vi "Submit Goal.vi"(8 "error in (no error)":errorcluster, 10 "Objective(s)":dbl[](array[numeric]) format="%#_13g", 11 "Generic Optimizer in":refnum<class "Generic Optimizer.lvclass">) -> (0 "error out":errorcluster, 3 "Generic Optimizer out":refnum<class "Generic Optimizer.lvclass">)   [LabVIEW 2020, in "RxnRover.lvlib" / "Generic Optimizer.lvclass"]
uses:
  Generic Optimizer.lvclass
  Generic Optimizer.lvclass/Generic Optimizer.ctl
  <userlib>/RxnRover/DynamicReentrant/Dynamic Reentrant.lvlib
  <vilib>/ErrorRing/Error Ring.xnode
  <vilib>/Utility/error.llb/Error Cluster From Error Code.vi
  Controller/Generic Plugin.lvclass
  C:/Users/zachc/programs/rxnrover_workspace/projects/rxnrover_exe/rxnrover/src/RxnRover/Plugin Servers/Controller/Generic Plugin.lvclass
  C:/Users/zachc/programs/rxnrover_workspace/projects/rxnrover_exe/rxnrover/src/RxnRover/Plugin Servers/Generic Optimizer/Generic Optimizer.lvclass
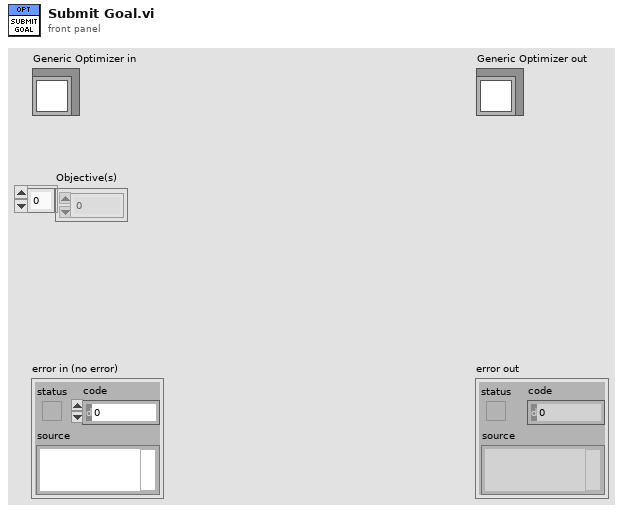
[diagram p1: front panel]
types:
  T1 = typedef "Dynamic Reentrant.lvlib/Message.ctl" = cluster{"Source":string, "Destination":string, "Time Stamp":timestamp, "Command":string, "Data":variant}
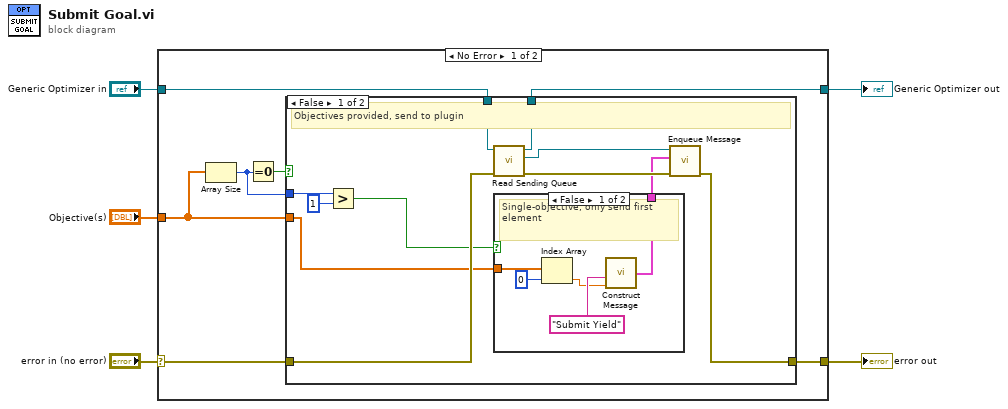
[diagram p0: block diagram]
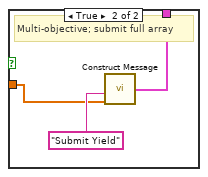
[diagram p2: hidden frame]
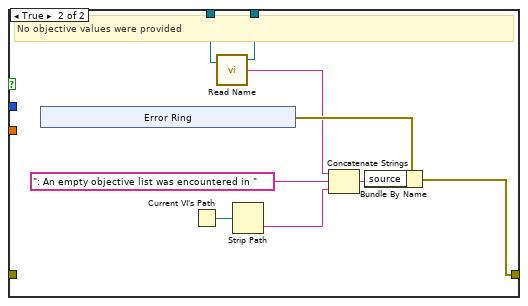
[diagram p3: hidden frame]
diagram:
  n1 = case shown="No Error" "error in (no error)" {
    selector: "error in (no error)" -> [w12 w46]
    tunnel: [w9 w46] -> w4
    tunnel: [w10 w45] -> w2
    tunnel: "Generic Optimizer in" -> [w11 w45]
    tunnel: "Objective(s)" -> [w7 _]
    frame No Error {
      n2 = Array Size(array=w7) -> (size(s)=w6:i32)
      n3 = Equal To 0?(x=w6) -> (x = 0?=w8:bool)
      n4 = case shown="False" w8 {
        tunnel: w12 -> [w23 _]
        tunnel: w11 -> [w22 w40]
        tunnel: [w21 w38] -> w10
        tunnel: [w17 w32] -> w9
        tunnel: w7 -> [w13 _]
        tunnel: w6 -> [w16 _]
        frame False {
          # "Objectives provided, send to plugin"
          n5 = Greater?(x=w16, y=1) -> (0:w14:bool)
          n6 = call-dynamic "Read Sending Queue.vi"("error in (no error)"=w23, "Generic Controller in"=w22) -> ("error out"=w20:errorcluster, "Sending Queue"=w19:refnum<queue>, "Generic Controller out"=w21:refnum<class "Generic Optimizer.lvclass">)  [unwired: 7 in]
          n7 = case shown="False" w14 {
            tunnel: [w27 w30] -> w18
            tunnel: w13 -> [w26 w29]
            frame False {
              # "Single-objective; only send first element"
              n8 = Index Array(array=w26, index=0) -> (element=w24:dbl)
              n9 = call <userlib>:"Construct Message.vi"("Data"=w24, "Command"="Submit Yield") -> ("Message Cluster"=w27:T1)  [unwired: 4 in]
            }
            frame True {
              # "Multi-objective; submit full array"
              n10 = call <userlib>:"Construct Message.vi"("Data"=w29, "Command"="Submit Yield") -> ("Message Cluster"=w30:T1)  [unwired: 4 in]
            }
          }
          n11 = call <userlib>:"Enqueue Message.vi"("error in (no error)"=w20, "Message"=w18, "Listening Queue"=w19) -> ("error out"=w17:errorcluster)  [unwired: 7 in, 1 out]
        }
        frame True {
          # "No objective values were provided"
          n12 = xnode "Error Ring"() -> ("error out"=w39:errorcluster)
          n13 = Current VI's Path() -> (path=w34:path)
          n14 = call "Read Name.vi"("controller in"=w40) -> ("controller out"=w38:refnum<class "Generic Optimizer.lvclass">, "Name"=w36:string)  [unwired: 1 in, 1 out]
          n15 = Strip Path(path=w34) -> (name=w33:string)  [unwired: 1 out]
          n16 = Concatenate Strings(w36, ": An empty objective list was encountered in " ("source"), w33) -> (w37:string)
          n17 = Bundle By Name(cluster=w39, "source"=w37) -> (w32:errorcluster)
        }
      }
    }
    frame Error {
    }
  }
  "error out" <- w4
  "Generic Optimizer out" <- w2
